vi "Server_Channels_Kernal.vi"(0 "Board type":T2=enum."NB-MIO-16H", 1 "interval scanning":bool, 2 "Client Time":dbl, 5 "No of samples+extra":i32=128 min=0 step=1, 7 "Trigger mode":T1, 9 "output polarity":u16(ring)=1 items=["do not change", "positive", "negative"], 11 "Ch & spans":T3[](array[typedef]) {"low limit (-10V)" format="%.3f"; "high limit (10V)" format="%.3f"}, 12 "Actual Sampling rate (Hz)":dbl=1000.0 format="%.2f", 13 "Local Client?":bool, 14 "Current Block No":i32) -> (4 "I16 data":i16[][](array[numeric]), 6 "Block Timings":T4={"Started"=0.0, "Ended"=0.0, "Analogue Frequency Hz"=1000.0} {"Analogue Frequency Hz" format="%.2f"}, 10 "group channel settings":T5(array[cluster]) {"scale offset" format="%.2f"; "scale multiplier" format="%.2f"; "gain" format="%.2f"; "range" format="%.2f"; "lower input limits" format="%.2f"; "upper input limits" format="%.2f"}, 15 "error out":errorcluster)   [LabVIEW 2010]
uses:
  Controls/Block_start_and_end.ctl
  Controls/Ch_and_Spans.ctl
  Controls/Board_Types.ctl
  Controls/Trigger_Mode.ctl
  ADAM Client/Sub VIs/ADAM Controls/Search_mode.ctl
  Globals/Trav_pos_global.vi
  Globals/Meas_global.vi
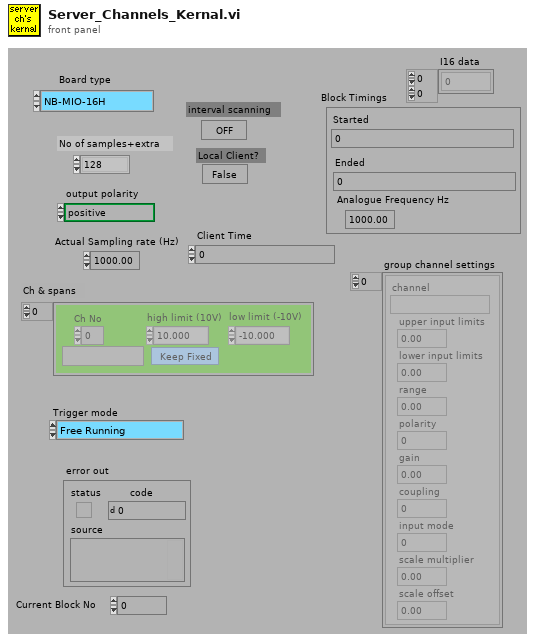
[diagram p1: front panel]
types:
  T1 = typedef "Trigger_Mode.ctl" = enum16{"Free Running", "Start on Trigger", "Trigger Every Block", "Trigger Every Sample"}
  T2 = typedef "Board_Types.ctl" = enum16{"Simulate", "NB-MIO-16H", "PCI-MIO-16E", "6000E Series", "USB-92xx", "ADC488", "Lab-NB", "NB-DIO-24", "NI-DAQmx", "Local ADAM", "Server Channels"}
  T3 = typedef "Ch_and_Spans.ctl" = cluster{"high limit (10V)":sgl, "low limit (-10V)":sgl, "Ch No":i16, "Var name":string, "Use Latest Calib":bool}
  T4 = typedef "Block_start_and_end.ctl" = cluster{"Started":dbl, "Ended":dbl, "Analogue Frequency Hz":dbl}
  T5 = cluster{"channel":string, "upper input limits":sgl, "lower input limits":sgl, "range":sgl, "polarity":u16, "gain":sgl, "coupling":u16, "input mode":u16, "scale multiplier":dbl, "scale offset":dbl}[]
  T6 = typedef "Traverse_cluster.ctl" = cluster{"Start X":dbl, "Start Y":dbl, "Start Z":dbl, "End X":dbl, "End Y":dbl, "End Z":dbl, "No. of pts.":i32, "Spacing":T7, "Filename":path, "Tunnel Speed":dbl, "Averaging time (min)":dbl, "Extra Commands":string, "Specific Arguments":string, "Emission Rate (l/min)":dbl, "Trace Gas Concentration (%)":dbl, "Density Ratio":string, "Comments":string, "Row No":i32, "Row Type Selector":T8, "Completion time":string, "Row Duration (mins)":dbl, "No. of Valid pts.":i32, "Meas Setup File":string}
  T7 = typedef "Spacing.ctl" = enum16{"Linear", "Log", "Gauss", "Specified", "N/A"}
  T8 = typedef "Multi_run_mode.ctl" = enum16{"Move Traverse Only", "Set Tunnel Speed Only", "Set Source Only", "Set Measurement Conditions", "Single Measurement", "Vertical Profile", "Lateral Profile", "Longitudinal Profile", "Explore Volume", "Multi-Axis Profile", "Auto Calibrate", "Meas Fast FID Bkgnd", "Check Beam Power", "Scanning Valve Measurement", "Run VI Named:", "Set ADAM Ch", "Wait (minutes)", "Send Message", "Synchronize With:", "Fall Back to this Row", "Turn Off Row Repeating", "Blank Row"}
  T9 = typedef "Search_mode.ctl" = enum16{"Between times", "All Times"}
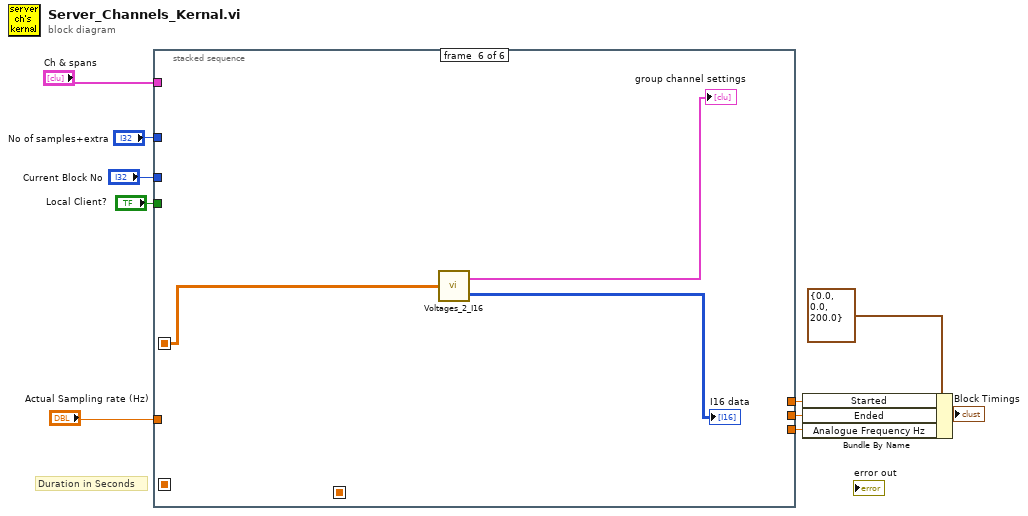
[diagram p0: block diagram]
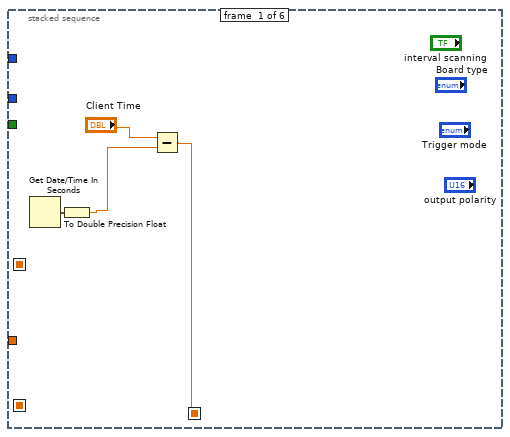
[diagram p2: hidden frame]
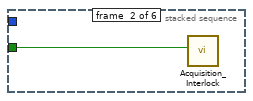
[diagram p3: hidden frame]
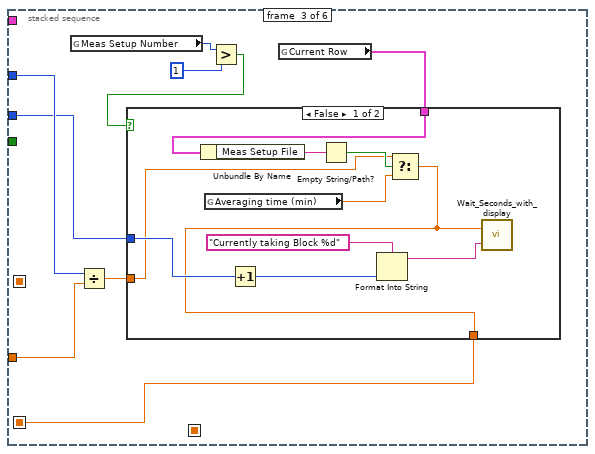
[diagram p4: hidden frame]
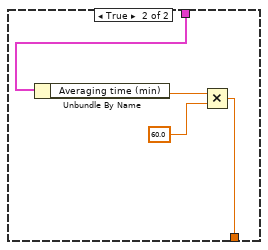
[diagram p5: hidden frame]
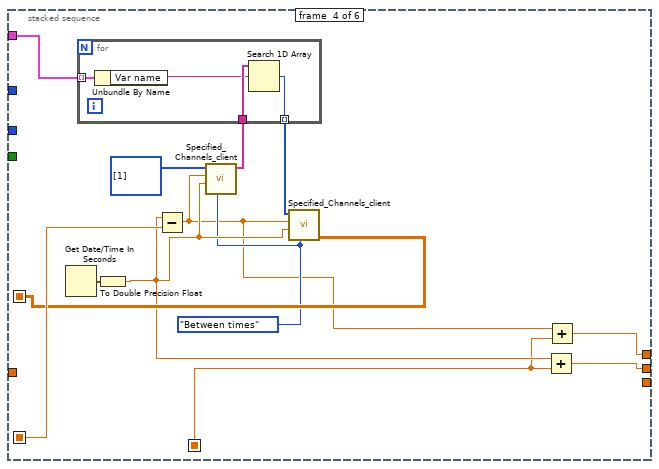
[diagram p6: hidden frame]
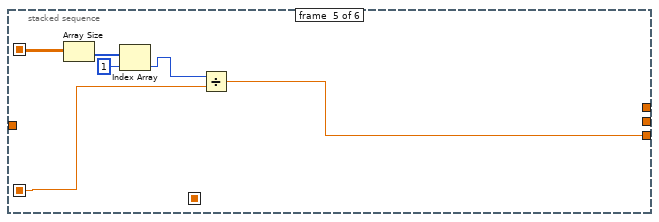
[diagram p7: hidden frame]
diagram:
  # "Duration in Seconds"
  n1 = stacked-sequence {
    seq-local: [_ _ _ w49 _ _] -> [_ _ _ _ w61 w62]
    seq-local: [w14 _ _ _ _ _] -> [_ _ _ w41 _ _]
    seq-local: [_ _ w20 _ _ _] -> [_ _ _ w50 w57 _]
    tunnel: "No of samples+extra" -> [_ _ w24 _ _ _]
    tunnel: "Current Block No" -> [_ _ w21 _ _ _]
    tunnel: [_ _ _ w39 _ _] -> w7
    tunnel: [_ _ _ w47 _ _] -> w6
    tunnel: "Local Client?" -> [_ w15 _ _ _ _]
    tunnel: "Ch & spans" -> [_ _ _ w48 _ _]
    tunnel: [_ _ _ _ w56 _] -> w2
    tunnel: "Actual Sampling rate (Hz)" -> [_ _ w23 _ _ _]
    frame #0 {
      n2 = Get Date/Time In Seconds() -> (seconds since 1Jan1904=w12:timestamp)
      n3 = To Double Precision Float(number=w12) -> (double precision float=w11:dbl)
      n4 = Subtract(x="Client Time", y=w11) -> (x-y=w14:dbl)
    }
    frame #1 {
      n5 = call "Acquisition_Interlock.vi"("Local Control"=w15) -> ()
    }
    frame #2 {
      n6 = global read "Trav_pos_global.vi" "Meas Setup Number"() -> (w18:i32)
      n7 = Divide(x=w24, y=w23) -> (x/y=w22:dbl)
      n8 = Greater?(x=w18, y=1) -> (0:w16:bool)
      n9 = global read "Trav_pos_global.vi" "Current Row"() -> (w19:T6)
      n10 = case shown="False" w16 {
        tunnel: w22 -> [w27 _]
        tunnel: w21 -> [w33 _]
        tunnel: [w26 w36] -> w20
        tunnel: w19 -> [w30 w35]
        frame False {
          n11 = Unbundle By Name(w30) -> ("Meas Setup File"=w29:string)
          n12 = global read "Meas_global.vi" "Averaging time (min)"() -> (w25:dbl)
          n13 = Increment(x=w33) -> (x+1=w31:i32)
          n14 = Empty String/Path?(string/path=w29) -> (empty?=w28:bool)
          n15 = Format Into String(format string="Currently taking Block %d" ("Message"), w31) -> (resulting string=w32:string)  [unwired: 2 in, 1 out]
          n16 = Select(t=w27, s=w28, f=w25) -> (s? t:f=w26:dbl)
          n17 = call "Wait_Seconds_with_display.vi"("Message"=w32, "Seconds to wait"=w26) -> ()  [unwired: 2 out]
        }
        frame True {
          n18 = Unbundle By Name(w35) -> ("Averaging time (min)"=w38:dbl)
          n19 = Multiply(x=w38, y=60.0) -> (x*y=w36:dbl)
        }
      }
    }
    frame #3 {
      w42 = Search_mode."Between times" ("Mode")
      n20 = Get Date/Time In Seconds() -> (seconds since 1Jan1904=w51:timestamp)
      n21 = To Double Precision Float(number=w51) -> (double precision float=w46:dbl)
      n22 = Subtract(x=w46, y=w50) -> (x-y=w40:dbl)
      n23 = call "Specified_Channels_client.vi"("Mode"=w42, "End time"=w46, "Start time"=w40, "ADAM Index array"=i32[] [1]) -> ("All Active Ch Names"=w44:string[])  [unwired: 1 in, 6 out]
      n24 = for {
        tunnel: w48 -> [w55] mode=indexing
        tunnel: w44 -> [w54]
        tunnel: [w52] -> w43 mode=indexing
        n25 = Unbundle By Name(w55) -> ("Var name"=w53:string)
        n26 = Search 1D Array(1D array=w54, element=w53) -> (index of element=w52:i32)  [unwired: 1 out]
      }
      n27 = call "Specified_Channels_client.vi"("Mode"=w42, "End time"=w46, "Start time"=w40, "ADAM Index array"=w43) -> ("Output array"=w49:dbl[][])  [unwired: 1 in, 6 out]
      n28 = Add(x=w46, y=w41) -> (x+y=w47:dbl)
      n29 = Add(x=w40, y=w41) -> (x+y=w39:dbl)
    }
    frame #4 {
      n30 = Array Size(array=w61) -> (size(s)=w60:i32[])
      n31 = Index Array(array=w60, index=1) -> (element=w58:i32)
      n32 = Divide(x=w58, y=w57) -> (x/y=w56:dbl)
    }
    frame #5 {
      n33 = call "Voltages_2_I16.vi"("Voltages"=w62) -> ("Group Channel Settings"=→"group channel settings":T5, "I16 data"=→"I16 data":i16[][])
    }
  }
  n34 = Bundle By Name(cluster=T4 {"Started"=0.0, "Ended"=0.0, "Analogue Frequency Hz"=200.0} ("Block Timings"), "Started"=w7, "Ended"=w6, "Analogue Frequency Hz"=w2) -> (→"Block Timings":T4)
